vi "WPI_UtilitiesFRC FPGATime.vi"(8 "error in (no error)":errorcluster) -> (0 "error out":errorcluster, 3 "FPGA Time":dbl)   [LabVIEW 2017]
doc: "Returns the current time reading of the clock on the FPGA image on the roboRIO device.\n\nThe <b>TimeStamp</b> parameter of the Interrupt Wait VI and the Direct Memory Access (DMA) stream both return the time on the clock.\n\nThis software is licensed. Open the labview\\readme\\WPI Robotics Library Open Source License.txt file for more information."
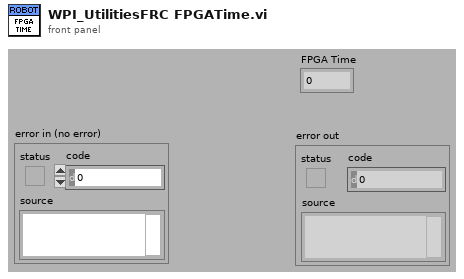
[diagram p1: front panel]
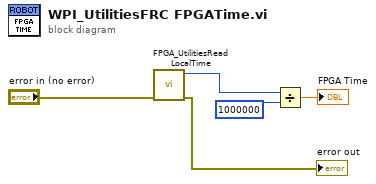
[diagram p0: block diagram]
diagram:
  n1 = call <vilib>:"FPGA_UtilitiesRead LocalTime.vi"("error in (no error)"="error in (no error)") -> ("error out"=→"error out":errorcluster, "LocalTime"=w5:u32)  [unwired: 9 out]
  n2 = Divide(x=w5, y=u32 1000000) -> (x/y=→"FPGA Time":dbl)
